vi "pythonsample.vi"() -> ()   [LabVIEW 2020]
panel:
  out "a + b":dbl
  in  "b":dbl=1.0
  in  "a":dbl=41.0
  in  "error in (no error)":errorcluster
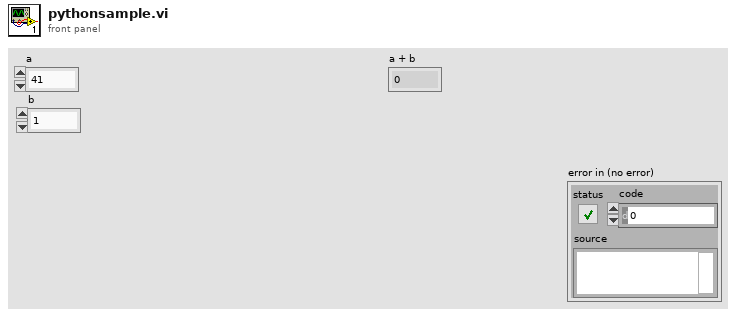
[diagram p1: front panel]
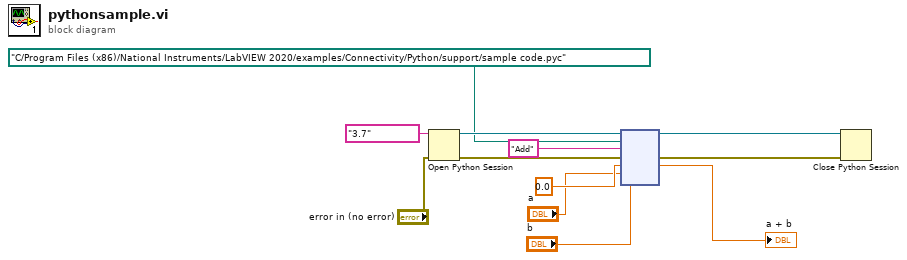
[diagram p0: block diagram]
diagram:
  n1 = Open Python Session(python version="3.7" ("Python version"), 3:"error in (no error)") -> (session out=w9:refnum<k35>, error out=w12:errorcluster)  [unwired: 1 in]
  n2 = node(w9, path "C:/Program Files (x86)/National Instruments/LabVIEW 2020/examples/Connectivity/Python/support/sample code.pyc" ("module path"), "Add" ("function name"), w12, 0.0 ("a"), "a", "b") -> (w11:refnum<k35>, w10:errorcluster, →"a + b":dbl)  [unwired: 2 in, 2 out]
  n3 = Close Python Session(session in=w11, error in=w10) -> ()  [unwired: 1 out]
